vi "Cartesian Transaction Lists.vi"(0 "Source":T1, 1 "Include Command":bool, 2 "error in (no error)":errorcluster) -> (3 "Cartesian Data":T2[](array[typedef]), 4 "Displacement Offsets":T2[](array[typedef]), 5 "Force Offsets":T2[](array[typedef]), 6 "error out":errorcluster)   [LabVIEW 2009]
uses:
  Dataset Transaction Id.ctl
  Dataset Source.ctl
  Dataset Type.ctl
  Apps/Yes No Button.ctl
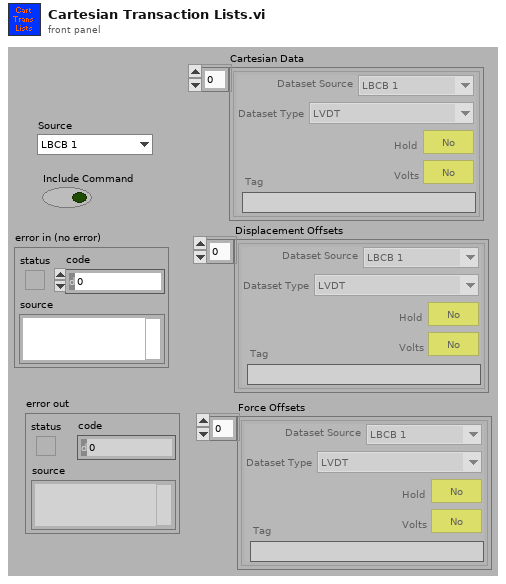
[diagram p1: front panel]
types:
  T1 = typedef "Dataset Source.ctl" = enum16{"LBCB 1", "LBCB 2", "Combined", "External Sensors"}
  T2 = typedef "Dataset Transaction Id.ctl" = cluster{"Dataset Source":T1, "Dataset Type":T3, "Hold":T4, "Volts":T4, "Tag":string}
  T3 = typedef "Dataset Type.ctl" = enum16{"LVDT", "Load Cell", "Actuator Command", "Servo Error", "Displacement Command", "Displacement", "Force"}
  T4 = typedef "Yes No Button.ctl" = bool
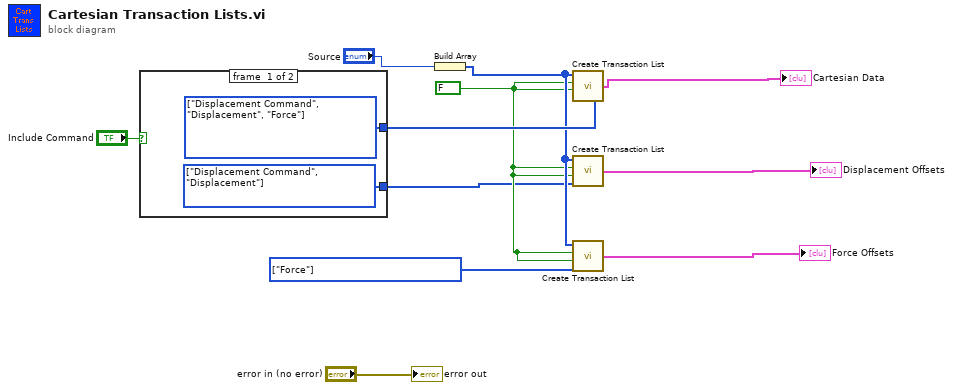
[diagram p0: block diagram]
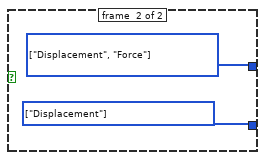
[diagram p2: hidden frame]
diagram:
  w3 = T3[] [enum."Force"] items=["LVDT", "Load Cell", "Actuator Command", "Servo Error", "Displacement Command", "Displacement", "Force"] ("Types")
  w5 = FALSE ("Volts")
  n1 = case shown="False" "Include Command" {
    tunnel: [w13 w15] -> w7
    tunnel: [w12 w14] -> w4
    frame #0 {
      w12 = T3[] [enum."Displacement Command", enum."Displacement"] items=["LVDT", "Load Cell", "Actuator Command", "Servo Error", "Displacement Command", "Displacement", "Force"] ("Types")
      w13 = T3[] [enum."Displacement Command", enum."Displacement", enum."Force"] items=["LVDT", "Load Cell", "Actuator Command", "Servo Error", "Displacement Command", "Displacement", "Force"] ("Types")
    }
    frame #1 {
      w14 = T3[] [enum."Displacement"] items=["LVDT", "Load Cell", "Actuator Command", "Servo Error", "Displacement Command", "Displacement", "Force"] ("Types")
      w15 = T3[] [enum."Displacement", enum."Force"] items=["LVDT", "Load Cell", "Actuator Command", "Servo Error", "Displacement Command", "Displacement", "Force"] ("Types")
    }
  }
  n2 = Build Array("Source") -> (w6:T1[])
  n3 = call "Create Transaction List.vi"("Types"=w7, "Hold"=w5, "Volts"=w5, "Sources"=w6) -> ("Transactions"=→"Cartesian Data":T2[])
  n4 = call "Create Transaction List.vi"("Types"=w4, "Hold"=w5, "Volts"=w5, "Sources"=w6) -> ("Transactions"=→"Displacement Offsets":T2[])
  n5 = call "Create Transaction List.vi"("Types"=w3, "Hold"=w5, "Volts"=w5, "Sources"=w6) -> ("Transactions"=→"Force Offsets":T2[])
  "error out" <- "error in (no error)"
